vi "test2.vi"() -> ()   [LabVIEW 2023]
uses:
  Devices/Flir A700/Flir A700.lvclass
  Camera Imaqdx/Configuration/Camera Imaqdx CFG.lvclass
  Camera Base/Camera Base.lvclass
  Devices/Rigol DS1054/Rigol DS1054.lvclass
  Devices/Rigol DS1054/Configurations/Fetch Display CFG/Fetch Display CFG.lvclass
  Camera Imaqdx/Camera Imaqdx.lvclass
  Scope/Scope Base/Scope Base.lvclass
  Camera Base/Acquisition Stats.ctl
panel:
  out "Last WF Mean":dbl
  out "Last Waveform":waveform(dbl)(graph)
  out "Acquisition Stats":T1
  out "Image":T2(plugin-control)
  out "error out cams":errorcluster
  out "error out scopes":errorcluster
  out "Error Out":errorcluster
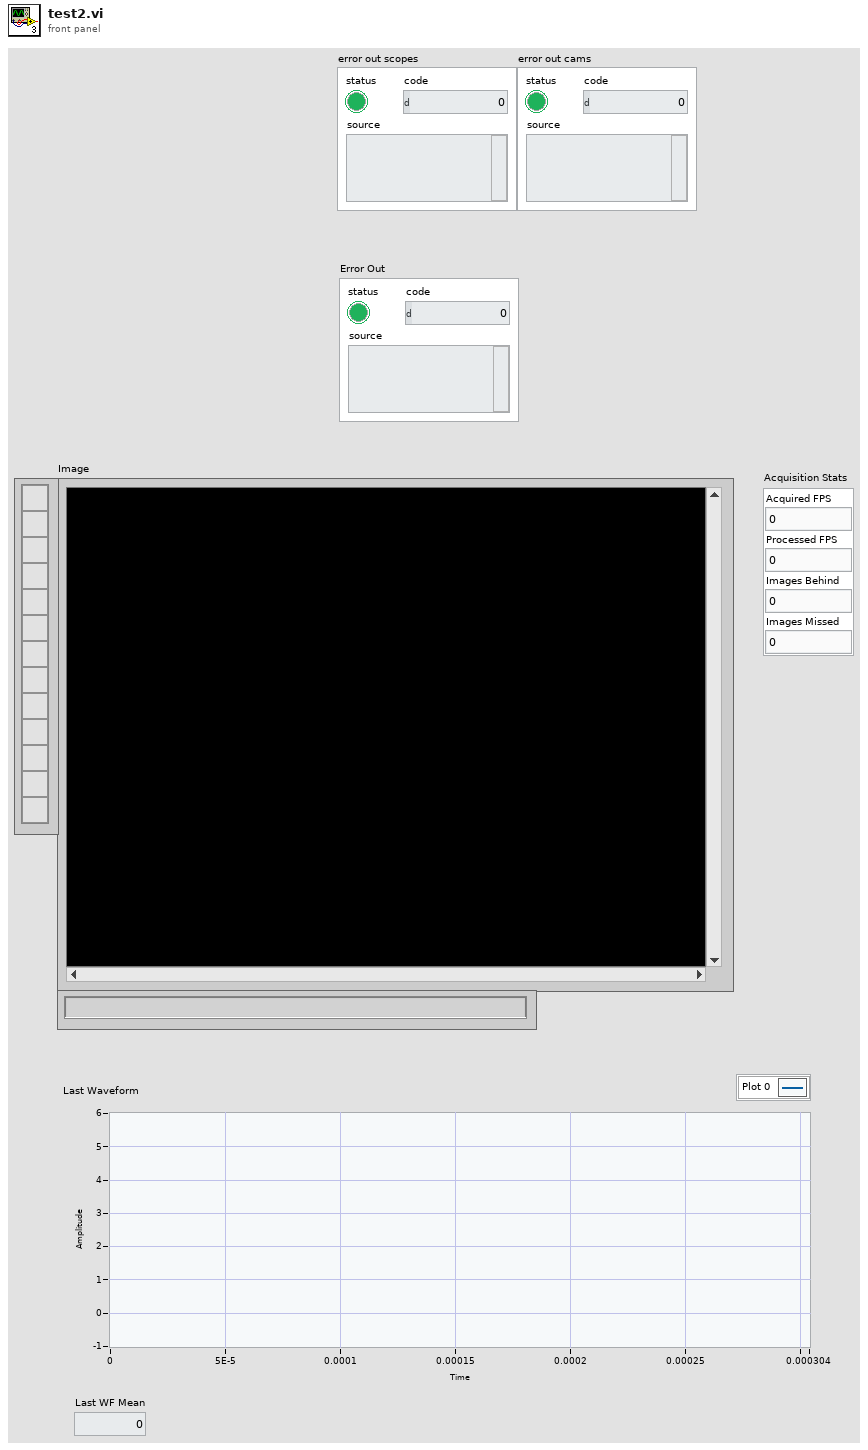
[diagram p1: front panel]
types:
  T1 = typedef "Camera.lvlib/Camera Base.lvclass/Acquisition Stats.ctl" = cluster{"Acquired FPS":dbl, "Processed FPS":dbl, "Images Behind":u32, "Images Missed":u32}
  T2 = typedef "IMAQ Image.ctl" = refnum<image>
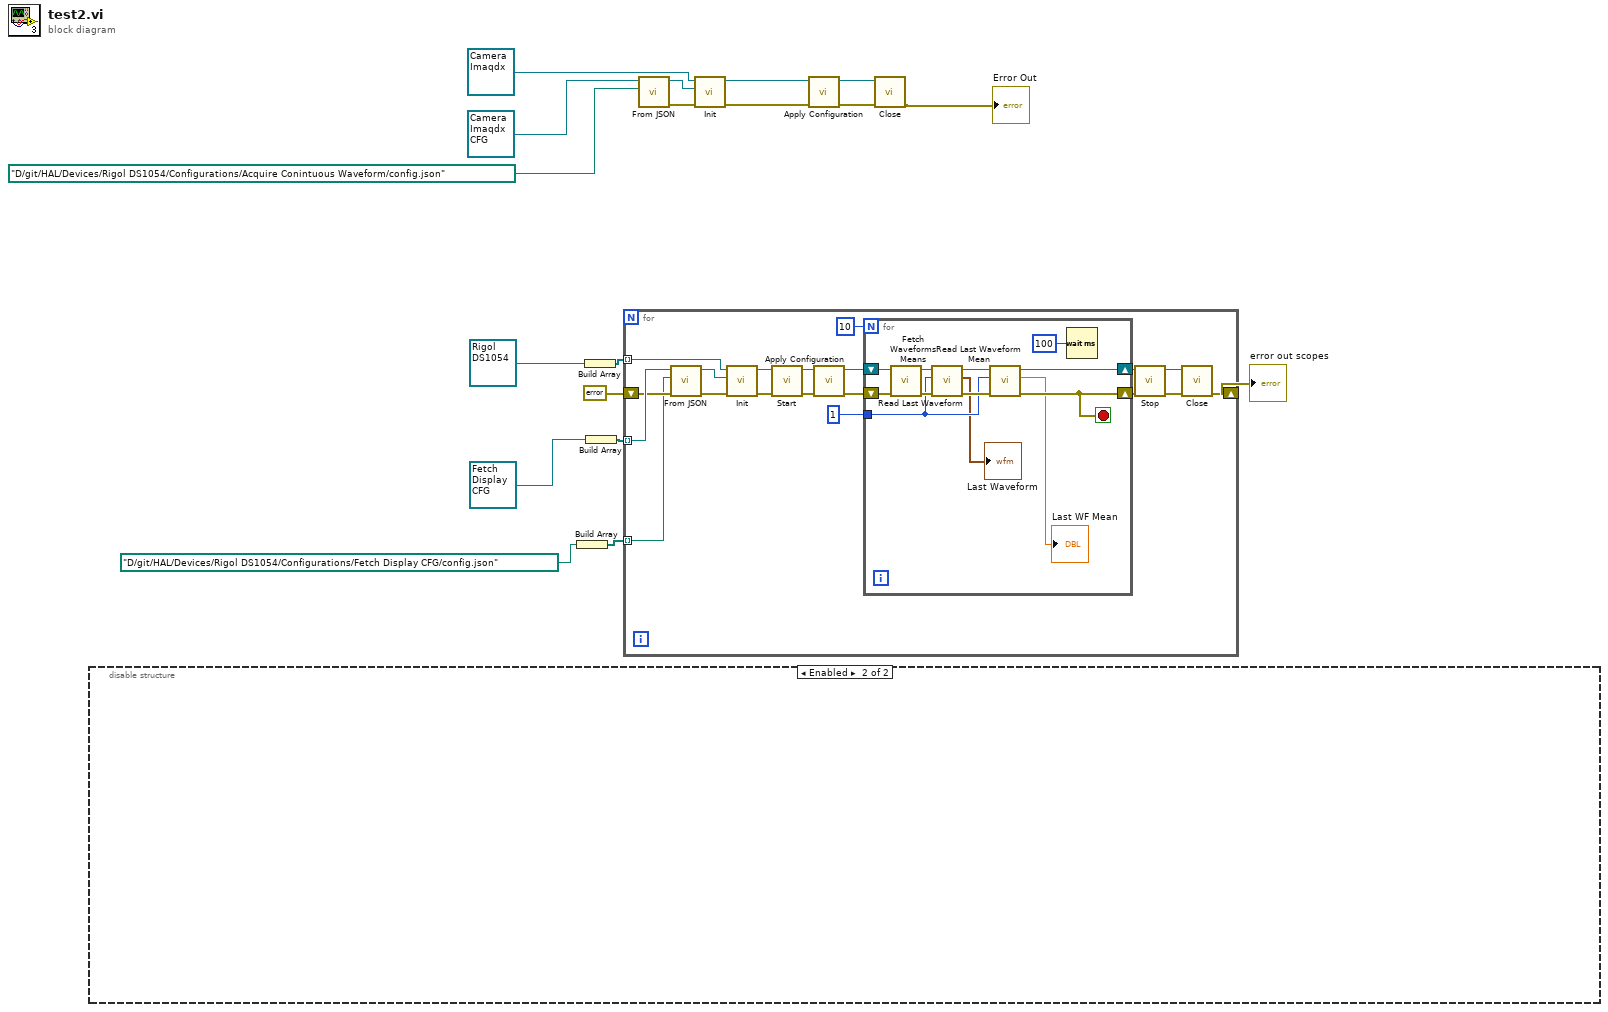
[diagram p0: block diagram]
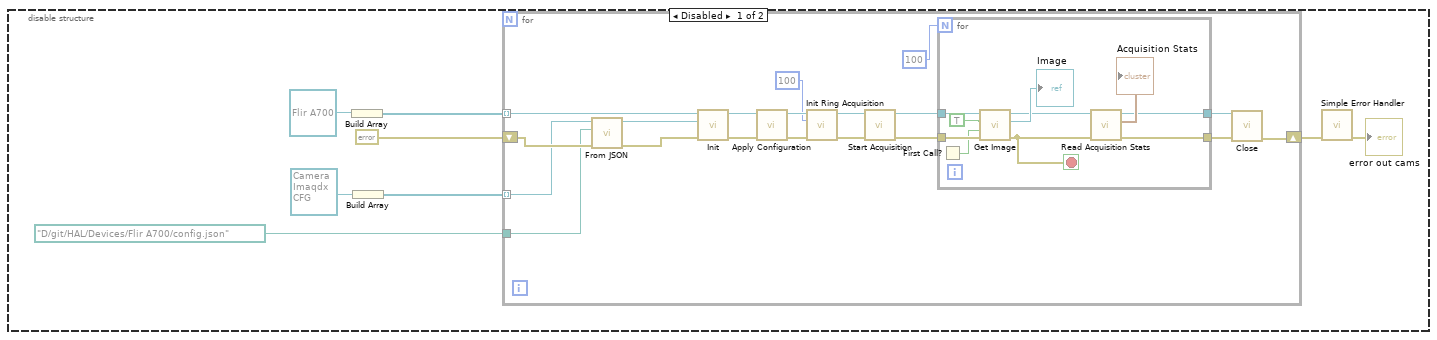
[diagram p2: hidden frame]
diagram:
  n1 = disable-structure shown="Enabled" {
    frame Disabled {
      n2 = Build Array(refnum<class "Flir A700.lvclass"> refnum ("FLIR A700.lvlib:Flir A700.lvclass")) -> (w23:refnum<class "Flir A700.lvclass">[])
      n3 = Build Array(refnum<class "Camera Imaqdx CFG.lvclass"> refnum ("HAL.lvlib:Camera Imaqdx CFG.lvclass")) -> (w24:refnum<class "Camera Imaqdx CFG.lvclass">[])
      n4 = for {
        tunnel: w23 -> [w45] mode=indexing
        tunnel: w24 -> [w39] mode=indexing
        shift-right: [w41] -> w26
        shift-left: errorcluster {"status"=FALSE, "code"=0, "source"=""} ("error constant") -> [w44]
        tunnel: path "D:/git/HAL/Devices/Flir A700/config.json" ("JSON Config") -> [w37]
        n5 = call-dynamic "From JSON.vi"("error in"=w44, "JSON Config"=w37, "object in"=w39) -> ("error out"=w40:errorcluster, "object out"=w38:refnum<class "Camera Imaqdx CFG.lvclass">)  [unwired: 7 in]
        n6 = call-dynamic "Init.vi"("error in (no error)"=w40, "IConfigure"=w38, "Flir A700 in"=w45) -> ("error out"=w43:errorcluster, "Flir A700 out"=w42:refnum<class "Flir A700.lvclass">)  [unwired: 7 in]
        n7 = call-dynamic "Apply Configuration.vi"("error in (no error)"=w43, "Camera Base in"=w42) -> ("error out"=w35:errorcluster, "Camera Base out"=w34:refnum<class "Flir A700.lvclass">)  [unwired: 8 in]
        n8 = call-dynamic "Init Ring Acquisition.vi"("error in (no error)"=w35, "Ring Buffer Size"=u32 100, "Camera Imaqdx in"=w34) -> ("error out"=w32:errorcluster, "Camera Imaqdx out"=w31:refnum<class "Flir A700.lvclass">)  [unwired: 7 in]
        n9 = call-dynamic "Start Acquisition.vi"("error in"=w32, "Camera Imaqdx in"=w31) -> ("error out"=w29:errorcluster, "Camera Imaqdx out"=w30:refnum<class "Flir A700.lvclass">)  [unwired: 8 in]
        n10 = for {
          N: 100 -> [_]
          tunnel: w30 -> [w54]
          tunnel: w29 -> [w55]
          tunnel: [w47] -> w28
          tunnel: [w46] -> w27
          stop <- w50 stop-if-true
          n11 = First Call?() -> (First Call?: T/F=w51:bool)
          n12 = call-dynamic "Get Image.vi"("error in"=w55, "Reset Stats?"=w51, "Calc Stats?"=TRUE, "Camera Imaqdx in"=w54) -> ("error out"=w50:errorcluster, "Image out"=→"Image":T2, "Camera Imaqdx out"=w48:refnum<class "Flir A700.lvclass">)  [unwired: 5 in]
          n13 = call "Read Acquisition Stats.vi"("error in (no error)"=w50, "Camera Base in"=w48) -> ("error out"=w47:errorcluster, "Acquisition Stats"=→"Acquisition Stats":T1, "Camera Base out"=w46:refnum<class "Flir A700.lvclass">)  [unwired: 7 in]
        }
        n14 = call-dynamic "Close.vi"("error in (no error)"=w28, "Camera Base in"=w27) -> ("error out"=w41:errorcluster)  [unwired: 8 in, 1 out]
      }
      n15 = call <vilib>:"Simple Error Handler.vi"("error in (no error)"=w26) -> ("error out"=→"error out cams":errorcluster)  [unwired: 4 in, 4 out]
    }
    frame Enabled {
    }
  }
  n16 = Build Array(path "D:/git/HAL/Devices/Rigol DS1054/Configurations/Fetch Display CFG/config.json" ("JSON Config")) -> (w12:path[])
  n17 = Build Array(refnum<class "Rigol DS1054.lvclass"> refnum ("RIGOL DS1054.lvlib:Rigol DS1054.lvclass")) -> (w18:refnum<class "Rigol DS1054.lvclass">[])
  n18 = Build Array(refnum<class "Fetch Display CFG.lvclass"> refnum ("RIGOL DS1054.lvlib:Continuous Waveform Acq CFG.lvclass")) -> (w17:refnum<class "Fetch Display CFG.lvclass">[])
  n19 = for {
    tunnel: w18 -> [w74] mode=indexing
    tunnel: w17 -> [w73] mode=indexing
    shift-right: [w71] -> w15
    shift-left: errorcluster {"status"=FALSE, "code"=0, "source"=""} ("error constant") -> [w69]
    tunnel: w12 -> [w67] mode=indexing
    n20 = call-dynamic "From JSON.vi"("error in (no error)"=w69, "JSON Config"=w67, "object in"=w73) -> ("error out"=w68:errorcluster, "object out"=w70:refnum<class "Fetch Display CFG.lvclass">)  [unwired: 7 in]
    n21 = call-dynamic "Init.vi"("Error In"=w68, "IConfigure"=w70, "object in"=w74) -> ("Error Out"=w72:errorcluster, "object out"=w65:refnum<class "Rigol DS1054.lvclass">)  [unwired: 7 in]
    n22 = call-dynamic "Start.vi"("Error In"=w72, "object in"=w65) -> ("Error Out"=w66:errorcluster, "object out"=w64:refnum<class "Rigol DS1054.lvclass">)  [unwired: 8 in]
    n23 = call-dynamic "Apply Configuration.vi"("error in"=w66, "Scope Base in"=w64) -> ("error out"=w60:errorcluster, "Scope Base out"=w61:refnum<class "Rigol DS1054.lvclass">)  [unwired: 8 in]
    n24 = for {
      N: 10 -> [_]
      tunnel: u8 1 ("Channel") -> [w79]
      shift-right: [w80] -> w58
      shift-left: w61 -> [w85]
      shift-right: [w78] -> w59
      shift-left: w60 -> [w84]
      stop <- w78 stop-if-true
      n25 = call-dynamic "Fetch Waveforms Means.vi"("error in"=w84, "Scope Base in"=w85) -> ("error out"=w86:errorcluster, "Scope Base out"=w82:refnum<class "Rigol DS1054.lvclass">)  [unwired: 8 in]
      n26 = call-dynamic "Read Last Waveform.vi"("error in (no error)"=w86, "Channel"=w79, "Scope Base in"=w82) -> ("error out"=w83:errorcluster, "Last Waveform"=→"Last Waveform":waveform(dbl), "Scope Base out"=w81:refnum<class "Rigol DS1054.lvclass">)  [unwired: 6 in]
      n27 = call-dynamic "Read Last Waveform Mean.vi"("error in (no error)"=w83, "Channel"=w79, "Scope Base in"=w81) -> ("error out"=w78:errorcluster, "Waveform Mean"=→"Last WF Mean":dbl, "Scope Base out"=w80:refnum<class "Rigol DS1054.lvclass">)  [unwired: 6 in]
      n28 = Wait (ms)(milliseconds to wait=u32 100) -> ()  [unwired: 1 out]
    }
    n29 = call-dynamic "Stop.vi"("Error In"=w59, "object in"=w58) -> ("Error Out"=w63:errorcluster, "object out"=w62:refnum<class "Rigol DS1054.lvclass">)  [unwired: 8 in]
    n30 = call-dynamic "Close.vi"("Error In"=w63, "object in"=w62) -> ("Error Out"=w71:errorcluster)  [unwired: 8 in, 1 out]
  }
  "error out scopes" <- w15
  n31 = call-dynamic "From JSON.vi"("JSON Config"=path "D:/git/HAL/Devices/Rigol DS1054/Configurations/Acquire Conintuous Waveform/config.json" ("File Path"), "object in"=refnum<class "Camera Imaqdx CFG.lvclass"> refnum ("Camera Imaqdx CFG.lvclass")) -> ("error out"=w3:errorcluster, "object out"=w10:refnum<class "Camera Imaqdx CFG.lvclass">)  [unwired: 8 in]
  n32 = call-dynamic "Init.vi"("error in (no error)"=w3, "IConfigure"=w10, "Camera Base in"=refnum<class "Camera Imaqdx.lvclass"> refnum ("Camera Imaqdx.lvclass")) -> ("error out"=w7:errorcluster, "Camera Base out"=w8:refnum<class "Camera Imaqdx.lvclass">)  [unwired: 7 in]
  n33 = call-dynamic "Apply Configuration.vi"("error in"=w7, "Scope Base in"=w8) -> ("error out"=w5:errorcluster, "Scope Base out"=w6:refnum<class "Scope Base.lvclass">)  [unwired: 8 in]
  n34 = call-dynamic "Close.vi"("Error In"=w5, "object in"=w6) -> ("Error Out"=→"Error Out":errorcluster)  [unwired: 8 in, 1 out]
